vi "read counter1.vi"(8 "error in (no error)":errorcluster, 11 "Waveform in":refnum<class "Waveform.lvclass">) -> (0 "error out":errorcluster, 3 "Waveform out":refnum<class "Waveform.lvclass">)   [LabVIEW 2012, in "Waveform.lvclass"]
uses:
  Waveform.lvclass
  Waveform.lvclass/Waveform.ctl
  <vilib>/DAQmx/read.llb/DAQmx Read (Counter 1D U32 1Chan NSamp).vi
  <vilib>/DAQmx/miscellaneous.llb/DAQmx Fill In Error Info.vi
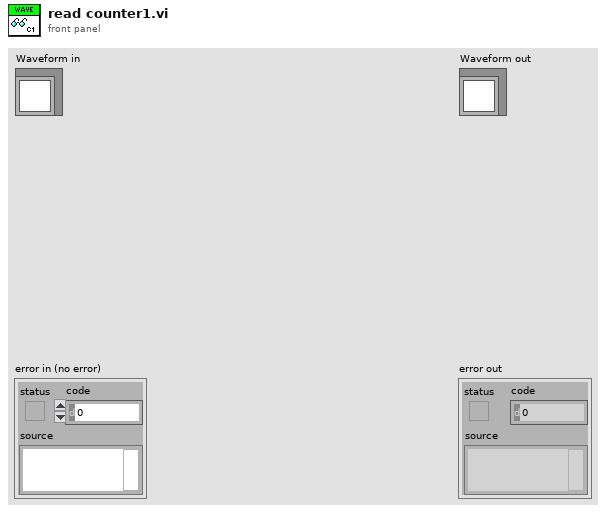
[diagram p1: front panel]
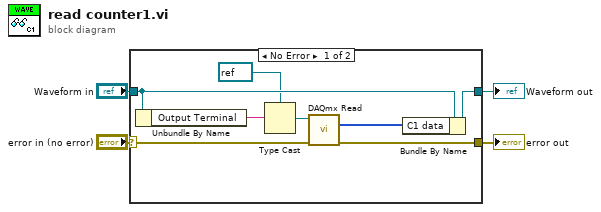
[diagram p0: block diagram]
diagram:
  n1 = case shown="No Error" "error in (no error)" {
    selector: "error in (no error)" -> [w12 w14]
    tunnel: [w11 w14] -> w3
    tunnel: [w9 w13] -> w1
    tunnel: "Waveform in" -> [w10 w13]
    frame No Error {
      n2 = Unbundle By Name(w10) -> ("Output Terminal"=w5:string)
      n3 = Type Cast(type=refnum<k21> refnum ("task/channels in"), x=w5) -> (*(type *) &x=w6:refnum<k21>)
      n4 = call-poly <vilib>:"DAQmx Read.vi"("task/channels in"=w6, "error in"=w12) -> ("data"=w8:u32[], "error out"=w11:errorcluster)  [unwired: 11 in, 1 out]
      n5 = Bundle By Name(cluster=w10, "C1 data"=w8) -> (w9:refnum<class "Waveform.lvclass">)
    }
    frame Error {
    }
  }
  "error out" <- w3
  "Waveform out" <- w1
